vi "LWXPS_GetHashCode.vi"(3 "LabVIEW error IN":errorcluster, 5 "XPS Reference IN":refnum<k24>) -> (0 "LabVIEW error OUT":errorcluster, 1 "Returned error code":i32, 2 "XPS Reference OUT":refnum<k24>)   [LabVIEW 2014]
uses:
  D:/XPSQ8_LabView_Library/Development/Source/Dll/Newport.XPS.CommandInterface.dll
  Dll/Newport.XPS.CommandInterface.dll
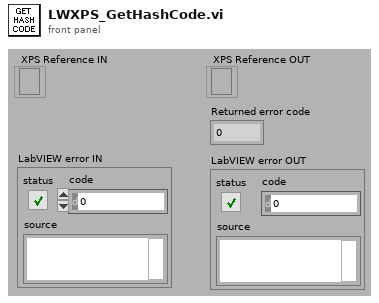
[diagram p1: front panel]
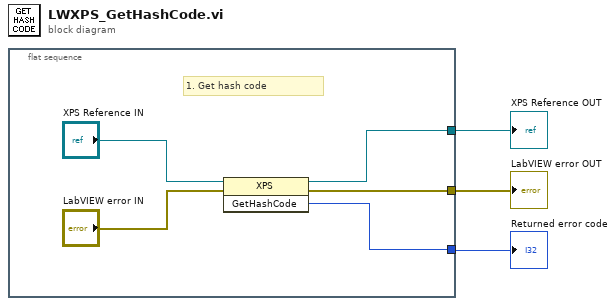
[diagram p0: block diagram]
diagram:
  n1 = flat-sequence {
    tunnel: [w7] -> w3
    tunnel: [w6] -> w2
    tunnel: [w5] -> w1
    frame #0 {
      # "1. Get hash code"
      n2 = invoke class="XPS" method="GetHashCode"(reference="XPS Reference IN", error in="LabVIEW error IN") -> (reference out=w7:refnum<k24>, error out=w6:errorcluster, "GetHashCode"=w5:i32)  [unwired: 1 in]
    }
  }
  "XPS Reference OUT" <- w3
  "LabVIEW error OUT" <- w2
  "Returned error code" <- w1
